vi "NearGoalCriteria.vi"(8 "error in (no error)":errorcluster, 10 "Point":dbl[](array[numeric]), 11 "TestObjetive in":refnum<class "TestObjetive.lvclass">) -> (0 "error out":errorcluster, 2 "evaluation":dbl, 3 "TestObjetive out":refnum<class "TestObjetive.lvclass">)   [LabVIEW 2023, in "TestObjetive.lvclass"]
uses:
  TestObjetive.lvclass
  TestObjetive.lvclass/TestObjetive.ctl
  Game_class/Game.lvclass/Game.ctl
  Game_class/Read FieldRef.vi
  Field_class/Field.lvclass
  Utilities_class/Utilities.lvclass
  Game_class/Game.lvclass
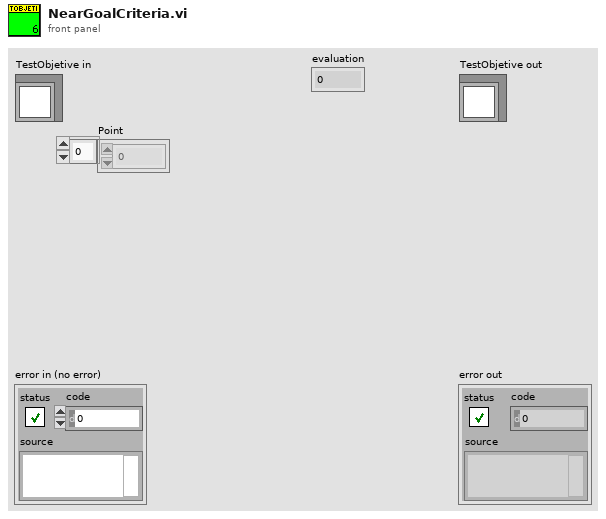
[diagram p1: front panel]
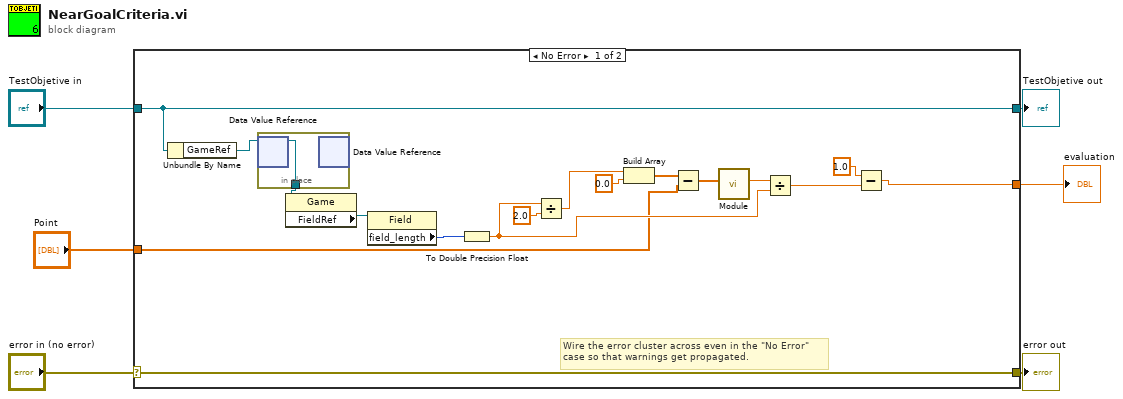
[diagram p0: block diagram]
diagram:
  n1 = case shown="No Error" "error in (no error)" {
    selector: "error in (no error)" -> [w23 w26]
    tunnel: [w23 w26] -> w5
    tunnel: [w14 w25] -> w3
    tunnel: "TestObjetive in" -> [w14 w25]
    tunnel: "Point" -> [w13 _]
    tunnel: [w7 _] -> w1
    frame No Error {
      # "Wire the error cluster across even in the \"No Error\"\ncase so that warnings get propagated."
      n2 = Unbundle By Name(w14) -> ("GameRef"=w12:refnum<data-value>)
      n3 = in-place {
        in-place-border: [w24] -> w11
        n4 = in-place-dvr #1(w12) -> (w24:refnum<class "Game.lvclass">)  [unwired: 1 out]
        n5 = in-place-dvr #1() -> ()  [unwired: 1 in, 2 out]
      }
      n6 = property class="Game"(reference=w11) -> ("FieldRef"=w10:refnum<class "Field.lvclass">)  [unwired: 1 in, 2 out]
      n7 = property class="Field"(reference=w10) -> ("field_length"=w9:i32)  [unwired: 1 in, 2 out]
      n8 = To Double Precision Float(number=w9) -> (double precision float=w15:dbl)
      n9 = Divide(x=w15, y=2.0) -> (x/y=w21:dbl)
      n10 = Build Array(w21, 0.0 ("element")) -> (w19:dbl[])
      n11 = Subtract(x=w19, y=w13) -> (x-y=w17:dbl[])
      n12 = call "Module.vi"("2D vector"=w17) -> ("Modulo"=w16:dbl)  [unwired: 8 in, 2 out]
      n13 = Divide(x=w16, y=w15) -> (x/y=w18:dbl)
      n14 = Subtract(x=1.0, y=w18) -> (x-y=w7:dbl)
    }
    frame Error {
    }
  }
  "error out" <- w5
  "TestObjetive out" <- w3
  "evaluation" <- w1
